vi "Pos ctrl window-Enqueue.vi"(8 "error in (no error)":errorcluster, 9 "variant":variant, 10 "States":T1, 11 "Pos ctrl window queue":refnum<queue>) -> (0 "error out":errorcluster)   [LabVIEW 2020]
uses:
  Typedefs/Pos Ctrl States.ctl
  Typedefs/Pos Ctrl queue data cluster.ctl
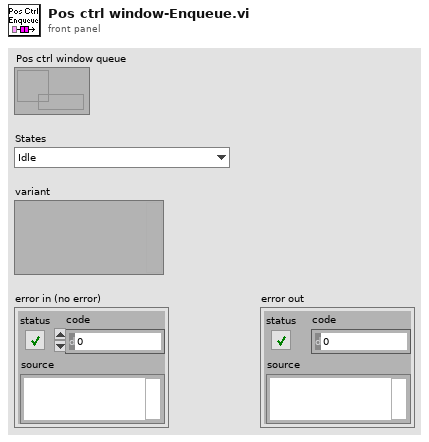
[diagram p1: front panel]
types:
  T1 = typedef "Pos Ctrl States.ctl" = enum16{"Idle", "Count-down", "Request single step (ack.)", "Request single step (no ack.)", "Request continuous movement", "Request movement stop"}
  T2 = typedef "Pos Ctrl queue data cluster.ctl" = cluster{"State":T1, "variant":variant}
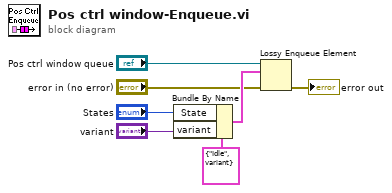
[diagram p0: block diagram]
diagram:
  n1 = Bundle By Name(cluster=T2 {"State"=enum."Idle", "variant"=variant} ("Pos Ctrl queue data cluster"), "State"="States", "variant"="variant") -> (w5:T2)
  n2 = Lossy Enqueue Element(queue="Pos ctrl window queue", element=w5, error in (no error)="error in (no error)") -> (error out=→"error out":errorcluster)  [unwired: 3 out]
